vi "Day4XYFromDirection.vi"(7 "Direction":T1, 10 "YIndex":i32, 11 "XIndex":i32) -> (2 "NewY":i32, 3 "NewX":i32)   [LabVIEW 2024]
uses:
  Day4Direction.ctl
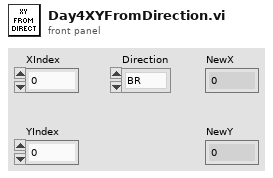
[diagram p1: front panel]
types:
  T1 = typedef "Day4Direction.ctl" = enum16{"BR", "BL", "B", "R", "L", "UR", "UL", "U"}
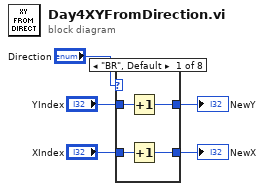
[diagram p0: block diagram]
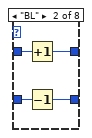
[diagram p2: hidden frame]
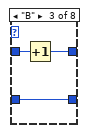
[diagram p3: hidden frame]
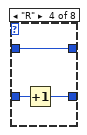
[diagram p4: hidden frame]
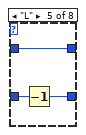
[diagram p5: hidden frame]
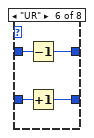
[diagram p6: hidden frame]
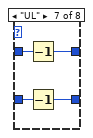
[diagram p7: hidden frame]
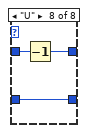
[diagram p8: hidden frame]
diagram:
  n1 = case shown="\"BR\", Default" "Direction" {
    tunnel: "XIndex" -> [w7 w13 w14 w19 w22 w26 w28 w31]
    tunnel: "YIndex" -> [w9 w12 w16 w17 w20 w24 w30 w33]
    tunnel: [w6 w11 w14 w18 w21 w25 w27 w31] -> w2
    tunnel: [w8 w10 w15 w17 w20 w23 w29 w32] -> w1
    frame "BR", Default {
      n2 = Increment(x=w9) -> (x+1=w8:i32)
      n3 = Increment(x=w7) -> (x+1=w6:i32)
    }
    frame "BL" {
      n4 = Increment(x=w12) -> (x+1=w10:i32)
      n5 = Decrement(x=w13) -> (x-1=w11:i32)
    }
    frame "B" {
      n6 = Increment(x=w16) -> (x+1=w15:i32)
    }
    frame "R" {
      n7 = Increment(x=w19) -> (x+1=w18:i32)
    }
    frame "L" {
      n8 = Decrement(x=w22) -> (x-1=w21:i32)
    }
    frame "UR" {
      n9 = Decrement(x=w24) -> (x-1=w23:i32)
      n10 = Increment(x=w26) -> (x+1=w25:i32)
    }
    frame "UL" {
      n11 = Decrement(x=w30) -> (x-1=w29:i32)
      n12 = Decrement(x=w28) -> (x-1=w27:i32)
    }
    frame "U" {
      n13 = Decrement(x=w33) -> (x-1=w32:i32)
    }
  }
  "NewX" <- w2
  "NewY" <- w1
